vi "ErrorCheckHWI.vi"(8 "error in (no error)":errorcluster, 11 "ArduinoDAC in":refnum<class "ArduinoDAC.lvclass">) -> (0 "error out":errorcluster, 3 "ArduinoDAC out":refnum<class "ArduinoDAC.lvclass">)   [LabVIEW 2013, in "ArduinoDAC.lvclass"]
uses:
  ArduinoDAC.lvclass
  ArduinoDAC.lvclass/ArduinoDAC.ctl
  <vilib>/Utility/error.llb/DialogType.ctl
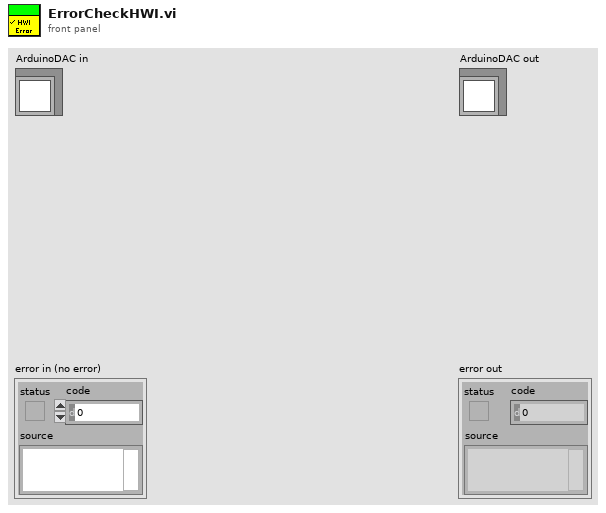
[diagram p1: front panel]
types:
  T1 = typedef "DialogType.ctl" = u16
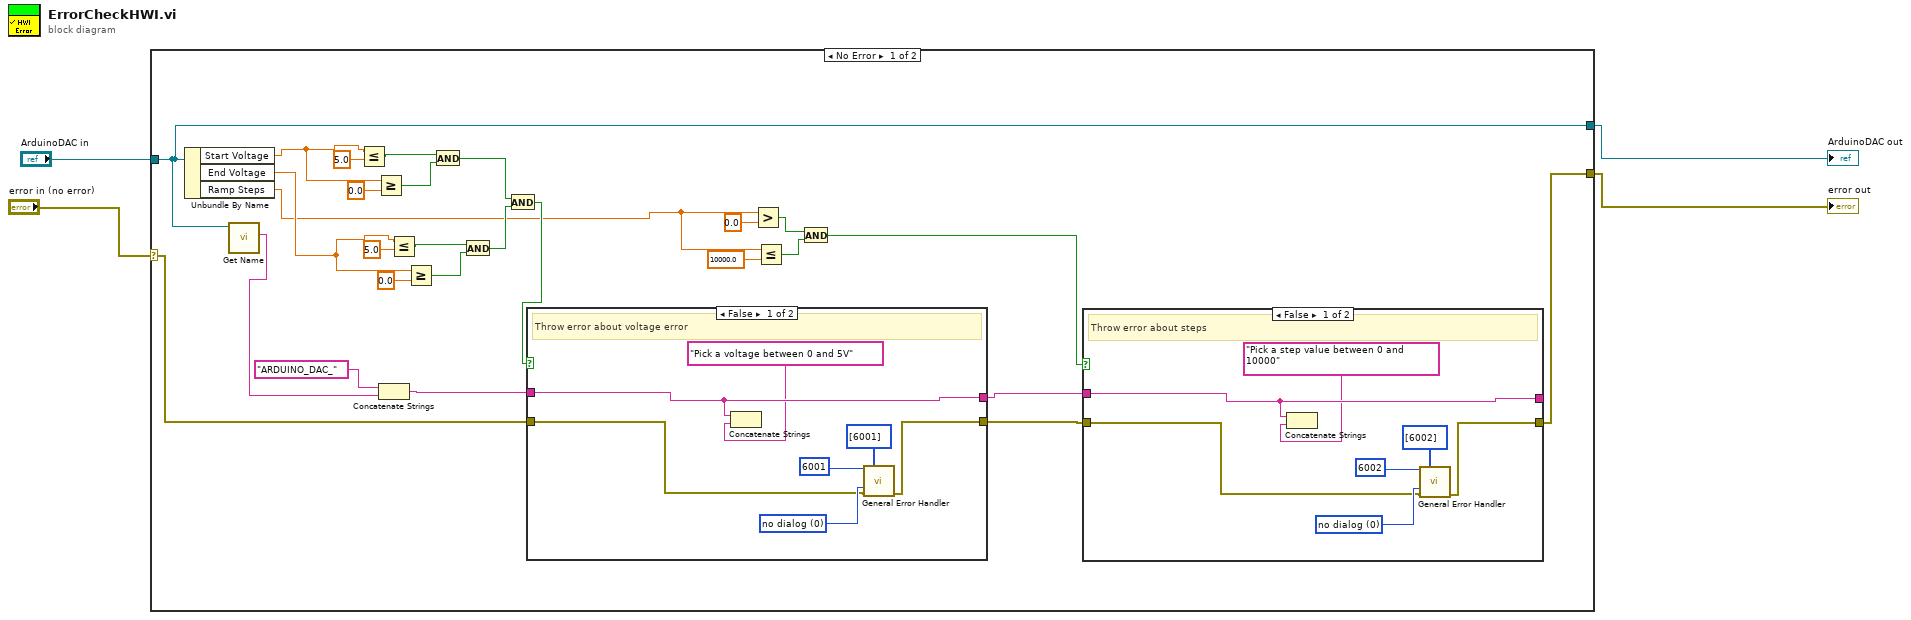
[diagram p0: block diagram]
diagram:
  n1 = case shown="No Error" "error in (no error)" {
    selector: "error in (no error)" -> [w17 w50]
    tunnel: "ArduinoDAC in" -> [w31 w51]
    tunnel: [w31 w51] -> w2
    tunnel: [w5 w50] -> w1
    frame No Error {
      n2 = Unbundle By Name(w31) -> ("Start Voltage"=w28:dbl, "End Voltage"=w21:dbl, "Ramp Steps"=w12:dbl)
      n3 = call-dynamic "Get Name.vi"("Device in"=w31) -> ("Name"=w15:string)  [unwired: 8 in, 2 out]
      n4 = Less Or Equal?(x=w28, y=5.0) -> (x <= y?=w30:bool)
      n5 = Greater Or Equal?(x=w28, y=0.0) -> (x >= y?=w26:bool)
      n6 = Concatenate Strings("ARDUINO_DAC_", w15) -> (w14:string)
      n7 = Less Or Equal?(x=w21, y=5.0) -> (x <= y?=w25:bool)
      n8 = Greater Or Equal?(x=w21, y=0.0) -> (x >= y?=w22:bool)
      n9 = And(x=w30, y=w26) -> (x .and. y?=w20:bool)
      n10 = And(x=w25, y=w22) -> (x .and. y?=w19:bool)
      n11 = And(x=w20, y=w19) -> (x .and. y?=w18:bool)
      n12 = case shown="False" w18 {
        tunnel: w17 -> [w46 w49]
        tunnel: w14 -> [w42 w48]
        tunnel: [w44 w49] -> w6
        tunnel: [w42 w48] -> w8
        frame False {
          w47 = T1 0 items=["no dialog", "OK message", "continue or stop message", "OK message + warnings", "continue/stop + warnings"] ("type of dialog (OK msg:1)")
          # "Throw error about voltage error"
          n13 = Concatenate Strings(w42, "Pick a voltage between 0 and 5V" ("format string")) -> ()  [unwired: 1 out]
          n14 = call <vilib>:"General Error Handler.vi"("[error code] (0)"=6001 ("error code (no error:0)"), "[user-defined codes]"=i32[] [6001], "type of dialog (OK msg:1)"=w47, "error in (no error)"=w46) -> ("error out"=w44:errorcluster)  [unwired: 7 in, 4 out]
        }
        frame True {
        }
      }
      n15 = Greater?(x=w12, y=0.0) -> (0:w9:bool)
      n16 = Less Or Equal?(x=w12, y=10000.0) -> (x <= y?=w10:bool)
      n17 = And(x=w9, y=w10) -> (x .and. y?=w7:bool)
      n18 = case shown="False" w7 {
        tunnel: w6 -> [w37 w40]
        tunnel: w8 -> [w33 w39]
        tunnel: [w35 w40] -> w5
        tunnel: [w33 w39] -> _
        frame False {
          w38 = T1 0 items=["no dialog", "OK message", "continue or stop message", "OK message + warnings", "continue/stop + warnings"] ("type of dialog (OK msg:1)")
          # "Throw error about steps"
          n19 = Concatenate Strings(w33, "Pick a step value between 0 and 10000" ("format string")) -> ()  [unwired: 1 out]
          n20 = call <vilib>:"General Error Handler.vi"("[error code] (0)"=6002 ("error code (no error:0)"), "[user-defined codes]"=i32[] [6002], "type of dialog (OK msg:1)"=w38, "error in (no error)"=w37) -> ("error out"=w35:errorcluster)  [unwired: 7 in, 4 out]
        }
        frame True {
        }
      }
    }
    frame Error {
    }
  }
  "error out" <- w1
  "ArduinoDAC out" <- w2
